vi "ReadFPBoolean.vi"(0 "FieldPoint IO Point Input":refnum<k21>) -> (1 "FieldPoint IO Point Output":refnum<k21>, 2 "Value":bool, 3 "timestamp":dbl format="%0.2f", 4 "error out":errorcluster)   [LabVIEW 2013]
uses:
  <vilib>/FieldPoint/Polymorphic Read.llb/FP Read (Boolean -IO).vi
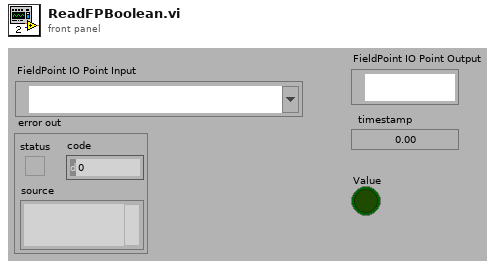
[diagram p1: front panel]
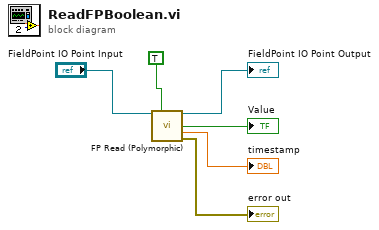
[diagram p0: block diagram]
diagram:
  n1 = call-poly <vilib>:"FP Read (Polymorphic).vi"("FieldPoint IO Point In"="FieldPoint IO Point Input", "Type"=TRUE) -> ("FieldPoint IO Point Out"=→"FieldPoint IO Point Output":refnum<k21>, "value"=→"Value":bool, "timestamp"=→"timestamp":dbl, "error out"=→"error out":errorcluster)  [unwired: 1 in, 9 out]
